vi "Type.vi"(11 "Type in":refnum<class "Type.lvclass">) -> (2 "Type":T1)   [LabVIEW 2020, in "Conditu2.lvlib" / "Columns.lvlib" / "Type.lvclass"]
uses:
  Type.lvclass
  Field Type.ctl
  Type.lvclass/Type.ctl
  Conditu2.lvlib
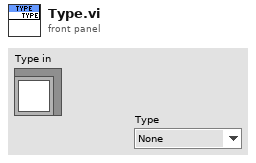
[diagram p1: front panel]
types:
  T1 = typedef "Conditu2.lvlib/Field Type.ctl" = enum16{"None", "ID", "Boolean", "Integer", "Double", "Timestamp", "String", "Text", "Entity"}
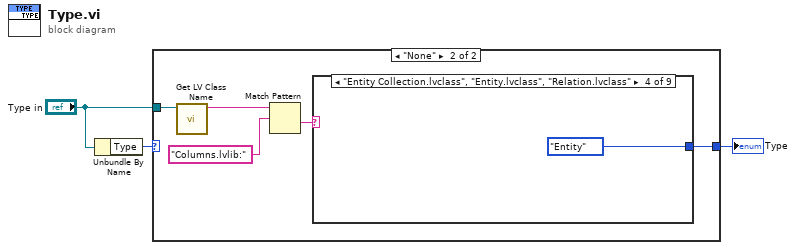
[diagram p0: block diagram]
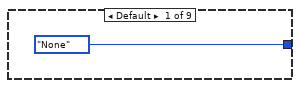
[diagram p3: hidden frame]
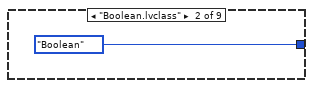
[diagram p4: hidden frame]
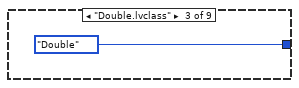
[diagram p5: hidden frame]
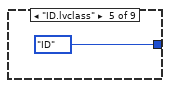
[diagram p6: hidden frame]
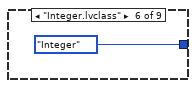
[diagram p7: hidden frame]
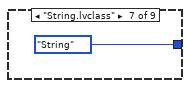
[diagram p8: hidden frame]
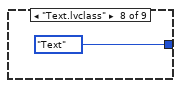
[diagram p9: hidden frame]
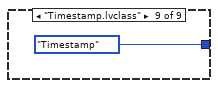
[diagram p10: hidden frame]
diagram:
  n1 = Unbundle By Name("Type in") -> ("Type"=w3:T1)
  n2 = case shown="\"None\"" w3 {
    selector: w3 -> [w4 _]
    tunnel: "Type in" -> [_ w9]
    tunnel: [w4 w5] -> w1
    frame Default {
    }
    frame "None" {
      n3 = call <vilib>:"Get LV Class Name.vi"("object"=w9) -> ("class name"=w8:string)  [unwired: 9 in, 1 out]
      n4 = Match Pattern(string=w8, regular expression="Columns.lvlib:") -> (after substring=w6:string)  [unwired: 1 in, 3 out]
      n5 = case shown="\"Entity Collection.lvclass\", \"Entity.lvclass\", \"Relation.lvclass\"" w6 {
        tunnel: [Field_Type."None" ("Type") Field_Type."Boolean" ("Type") Field_Type."Double" ("Type") Field_Type."Entity" ("Type") Field_Type."ID" ("Type") Field_Type."Integer" ("Type") Field_Type."String" ("Type") Field_Type."Text" ("Type") Field_Type."Timestamp" ("Type")] -> w5
        frame Default {
        }
        frame "Boolean.lvclass" {
        }
        frame "Double.lvclass" {
        }
        frame "Entity Collection.lvclass", "Entity.lvclass", "Relation.lvclass" {
        }
        frame "ID.lvclass" {
        }
        frame "Integer.lvclass" {
        }
        frame "String.lvclass" {
        }
        frame "Text.lvclass" {
        }
        frame "Timestamp.lvclass" {
        }
      }
    }
  }
  "Type" <- w1
